vi "Rio_Theta_Angle_To_Steps.vi"(9 "Current":i32, 10 "Desired":i32, 11 "Array in":i32[](array[numeric])) -> (3 "Array out":i32[](array[numeric]), 5 "Steps":dbl)   [LabVIEW 2017]
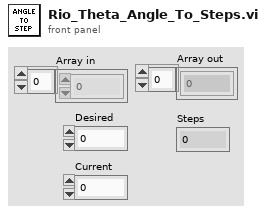
[diagram p1: front panel]
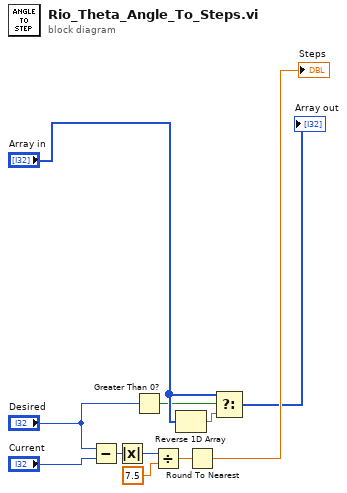
[diagram p0: block diagram]
diagram:
  n1 = Subtract(x="Desired", y="Current") -> (x-y=w5:i32)
  n2 = Absolute Value(x=w5) -> (abs(x)=w4:i32)
  n3 = Greater Than 0?(x="Desired") -> (x > 0?=w2:bool)
  n4 = Divide(x=w4, y=7.5) -> (x/y=w3:dbl)
  n5 = Reverse 1D Array(array="Array in") -> (reversed array=w1:i32[])
  n6 = Round To Nearest(number=w3) -> (nearest integer value=→"Steps":dbl)
  n7 = Select(t="Array in", s=w2, f=w1) -> (s? t:f=→"Array out":i32[])
